vi "test.vi"() -> ()   [LabVIEW 2019]
panel:
  out "Boolean":bool
  in  "stop 3":bool
  in  "stop 2":bool
  in  "stop":bool
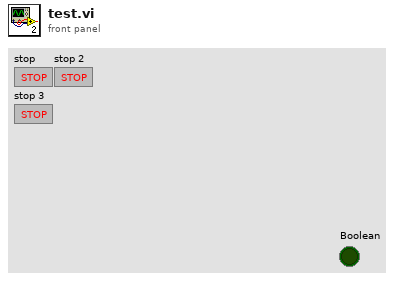
[diagram p1: front panel]
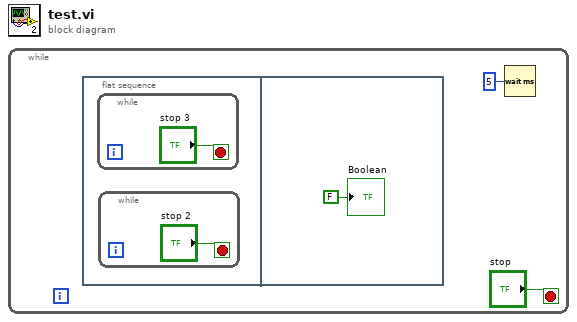
[diagram p0: block diagram]
diagram:
  n1 = while {
    stop <- "stop" stop-if-true
    n2 = flat-sequence {
      frame #0 {
        n3 = while {
          stop <- "stop 3" stop-if-true
        }
        n4 = while {
          stop <- "stop 2" stop-if-true
        }
      }
      frame #1 {
        "Boolean" <- FALSE ("Boolean")
      }
    }
    n5 = Wait (ms)(milliseconds to wait=u32 5) -> ()  [unwired: 1 out]
  }
